vi "_RT_Memory_Param.vi"(7 "Function":enum16{"Write", "Init", "Read"}(ring)=enum."Init", 8 "Error in":errorcluster, 10 "Data in":variant, 11 "Type of Var":T1) -> (0 "Error out":errorcluster, 3 "Data out":variant)   [LabVIEW 2016]
uses:
  PublicSubVI/ctl/_ctl_MassAnal_ParamType.ctl
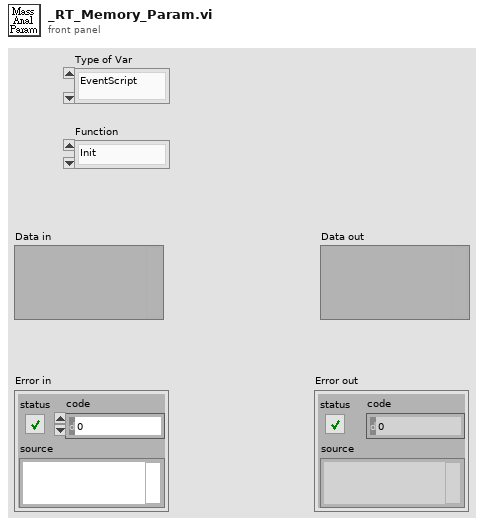
[diagram p1: front panel]
types:
  T1 = typedef "_ctl_MassAnal_ParamType.ctl" = enum16{"EventScript", "DO", "ExtAO"}
  T2 = enum16{"open", "replace", "create", "open or create", "replace or create", "replace or create with confirmation"}
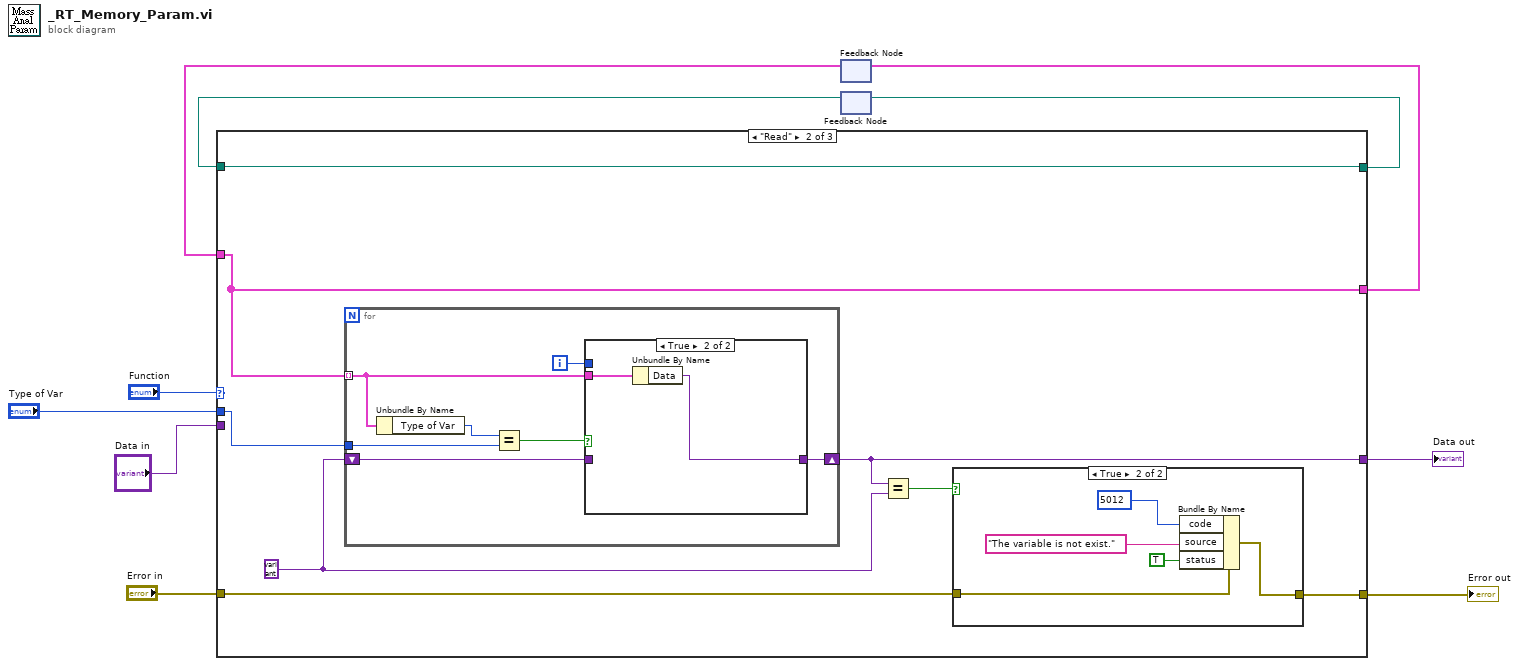
[diagram p0: block diagram]
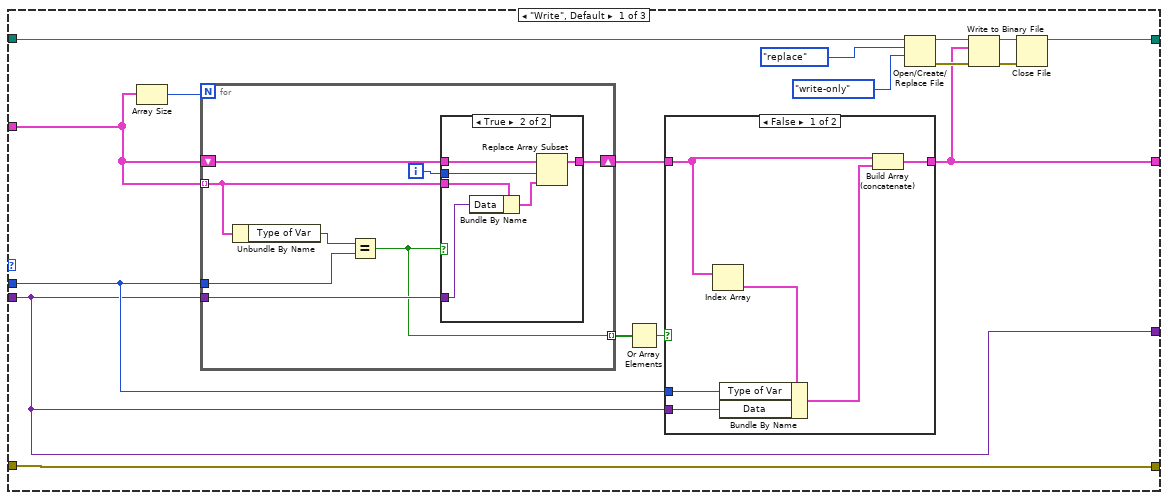
[diagram p2: hidden frame]
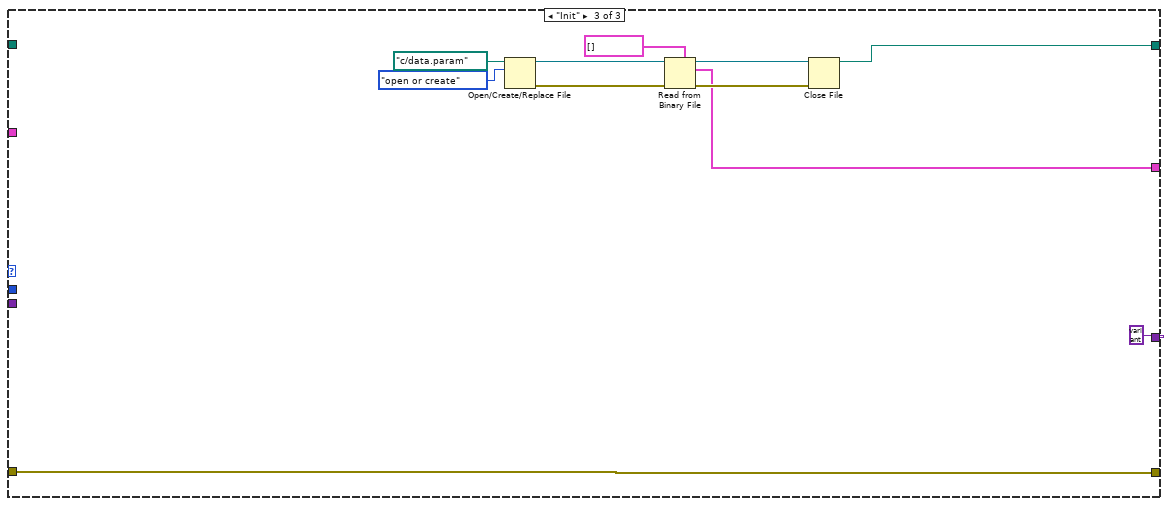
[diagram p7: hidden frame]
diagram:
  n1 = feedback #1() -> (w5:cluster{"Data":variant, "Type of Var":T1}[])  [unwired: 1 in]
  n2 = feedback #2() -> (w1:path)  [unwired: 1 in]
  n3 = case shown="\"Read\"" "Function" {
    tunnel: "Type of Var" -> [w23 w56 _]
    tunnel: "Data in" -> [w20 _ _]
    tunnel: "Error in" -> [w21 w53 w83]
    tunnel: [w21 w52 w83] -> w8
    tunnel: [w20 w55 variant ("Variant")] -> w6
    tunnel: w5 -> [w26 w57 _]
    tunnel: [w15 w57 w74] -> w4
    tunnel: [w11 w50 w76] -> w2
    tunnel: w1 -> [w18 w50 _]
    frame "Write", Default {
      n4 = Array Size(array=w26) -> (size(s)=w27:i32)
      n5 = for {
        N: w27 -> [_]
        tunnel: w26 -> [w39] mode=indexing
        tunnel: w23 -> [w41]
        tunnel: w20 -> [w40]
        shift-right: [w36] -> w22
        shift-left: w26 -> [w38]
        tunnel: [w35] -> w25 mode=indexing
        i -> [w37]
        n6 = Unbundle By Name(w39) -> ("Type of Var"=w42:T1)
        n7 = Equal?(x=w42, y=w41) -> (x = y?=w35:bool)
        n8 = case shown="True" w35 {
          tunnel: w39 -> [_ w49]
          tunnel: w40 -> [_ w48]
          tunnel: w38 -> [w43 w47]
          tunnel: w37 -> [_ w45]
          tunnel: [w43 w44] -> w36
          frame False {
          }
          frame True {
            n9 = Bundle By Name(cluster=w49, "Data"=w48) -> (w46:cluster{"Data":variant, "Type of Var":T1})
            n10 = Replace Array Subset(array=w47, new element=w46, index=w45) -> (w44:cluster{"Data":variant, "Type of Var":T1}[])
          }
        }
      }
      n11 = Or Array Elements(Boolean array=w25) -> (logical OR=w24:bool)
      n12 = case shown="False" w24 {
        tunnel: w23 -> [w33 _]
        tunnel: w20 -> [w32 _]
        tunnel: w22 -> [w29 w34]
        tunnel: [w30 w34] -> w15
        frame False {
          n13 = Index Array(array=w29) -> (element=w28:cluster{"Data":variant, "Type of Var":T1})  [unwired: 1 in]
          n14 = Bundle By Name(cluster=w28, "Type of Var"=w33, "Data"=w32) -> (w31:cluster{"Data":variant, "Type of Var":T1})
          n15 = Build Array (concatenate)(w29, w31) -> (w30:cluster{"Data":variant, "Type of Var":T1}[])
        }
        frame True {
        }
      }
      n16 = Open/Create/Replace File(file path (use dialog)=w18, operation (0:open)=T2."replace", access (0:read/write)=enum16{"read/write", "read-only", "write-only"}."write-only") -> (refnum out=w14:refnum<file>, error out=w16:errorcluster)  [unwired: 3 in, 1 out]
      n17 = Write to Binary File(file (use dialog)=w14, data=w15, error in=w16) -> (refnum out=w12:refnum<file>, error out=w13:errorcluster)  [unwired: 3 in, 1 out]
      n18 = Close File(refnum=w12, error in=w13) -> (path=w11:path)  [unwired: 1 out]
    }
    frame "Read" {
      w51 = variant ("Data")
      n19 = for {
        tunnel: w57 -> [w67] mode=indexing
        tunnel: w56 -> [w69]
        shift-right: [w65] -> w55
        shift-left: w51 -> [w64]
        i -> [w66]
        n20 = Unbundle By Name(w67) -> ("Type of Var"=w70:T1)
        n21 = Equal?(x=w70, y=w69) -> (x = y?=w68:bool)
        n22 = case shown="True" w68 {
          tunnel: w67 -> [_ w73]
          tunnel: w66 -> [_ _]
          tunnel: [w71 w72] -> w65
          tunnel: w64 -> [w71 _]
          frame False {
          }
          frame True {
            n23 = Unbundle By Name(w73) -> ("Data"=w72:variant)
          }
        }
      }
      n24 = Equal?(x=w55, y=w51) -> (x = y?=w54:bool)
      n25 = case shown="True" w54 {
        tunnel: w53 -> [w58 w63]
        tunnel: [w58 w62] -> w52
        frame False {
        }
        frame True {
          n26 = Bundle By Name(cluster=w63, "code"=5012, "source"="The variable is not exist.", "status"=TRUE) -> (w62:errorcluster)
        }
      }
    }
    frame "Init" {
      n27 = Open/Create/Replace File(file path (use dialog)=path "c:/data.param", operation (0:open)=T2."open or create") -> (refnum out=w80:refnum<file>, error out=w79:errorcluster)  [unwired: 4 in, 1 out]
      n28 = Read from Binary File(5:cluster{"Data":variant, "Type of Var":T1}[] [], 8:w79, 11:w80) -> (0:w78:errorcluster, 2:w74:cluster{"Data":variant, "Type of Var":T1}[], 3:w77:refnum<file>)  [unwired: 3 in, 1 out]
      n29 = Close File(refnum=w77, error in=w78) -> (path=w76:path)  [unwired: 1 out]
    }
  }
  "Error out" <- w8
  "Data out" <- w6
  n30 = feedback-in #1(w4) -> ()
  n31 = feedback-in #2(w2) -> ()
